vi "usrp get rx lo freq.vi"(7 "rx_lo_freq_out":dbl, 8 "error in (no error)":errorcluster, 9 "chan":u64, 10 "name":string, 11 "h":u64) -> (0 "error out":errorcluster, 3 "function return":u32(ring), 5 "rx_lo_freq_out out":dbl)   [LabVIEW 2023, in "uhd.lvlib"]
doc: "UHD_API uhd_error uhd_usrp_get_rx_lo_freq(\n uhd_usrp_handle h, const char* name, size_t chan, double* rx_lo_freq_out);"
uses:
  <userlib>/uhd/uhd.lvlib
  <userlib>/uhd/uhd.dll
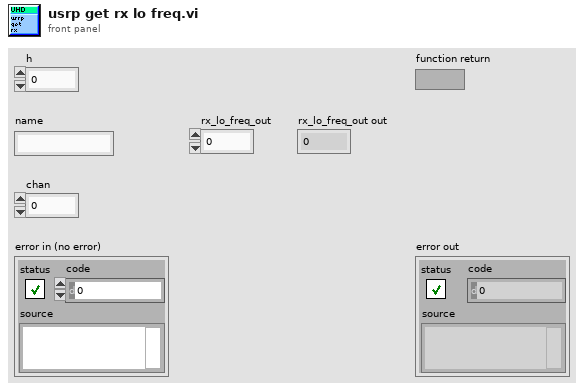
[diagram p1: front panel]
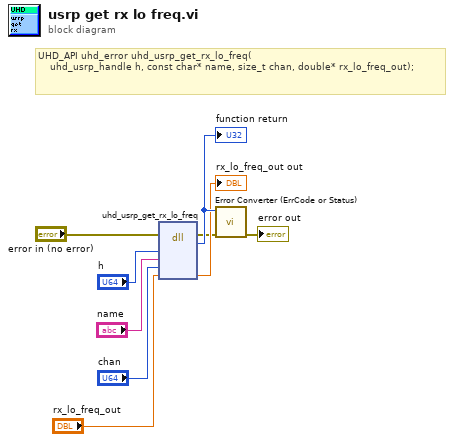
[diagram p0: block diagram]
diagram:
  # "UHD_API uhd_error uhd_usrp_get_rx_lo_freq(\n    uhd_usrp_handle h, const char* name, size_t chan, double* rx_lo_freq_out);"
  n1 = dll-call lib="C:/Program Files/National Instruments/LabVIEW 2023/user.lib/uhd/uhd.*" fn="uhd_usrp_get_rx_lo_freq"(error in="error in (no error)", "h"="h", "name"="name", "chan"="chan", "rx_lo_freq_out"="rx_lo_freq_out") -> (error out=w2:errorcluster, w9:u32, "rx_lo_freq_out"=→"rx_lo_freq_out out":dbl)  [unwired: 5 in, 1 out]
  "function return" <- w9
  n2 = call <userlib>:"Error Converter (ErrCode or Status).vi"("error in (no error)"=w2, "error code"=w9) -> ("error out"=→"error out":errorcluster)  [unwired: 9 in]
